vi "ConstantToArray_U64Color.vi"(11 "Constant":u64) -> (3 "ConstantArray":dbl[](array[numeric]))   [LabVIEW 2020, in "OpenLvVision_OpenCv.lvlib"]
uses:
  OpenLvVision_OpenCv.lvlib
  <vilib>/OpenLvVision/OpenLvVision_Image/DataAccess/OLV DataAccess.lvlib
  <vilib>/OpenLvVision/OpenLvVision_Image/DataAccess/NumberToColor/OLV U64toRgba.vi
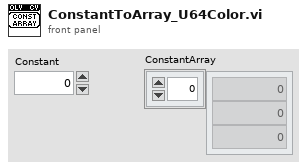
[diagram p1: front panel]
types:
  T1 = typedef "Color (U64)" = cluster{"Plane 3 (Blue)":u16, "Plane 2 (Green)":u16, "Plane 1 (Red)":u16, "Plane 4 (alpha)":u16}
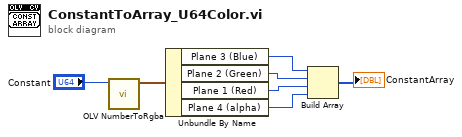
[diagram p0: block diagram]
diagram:
  n1 = call-poly <vilib>:"OLV NumberToRgba.vi"("U64"="Constant") -> ("Rgba"=w6:T1)  [unwired: 10 in]
  n2 = Unbundle By Name(w6) -> ("Plane 3 (Blue)"=w5:u16, "Plane 2 (Green)"=w4:u16, "Plane 1 (Red)"=w3:u16, "Plane 4 (alpha)"=w2:u16)
  n3 = Build Array(w5, w4, w3, w2) -> (→"ConstantArray":u16[])
